vi "Sequence for 3D calibration.vi"() -> ()   [LabVIEW 2011]
doc: "The Sequence VI acquires a sequence of images and displays the images in an image control using high-level acquisition VIs. A sequence is appropriate for applications in which you want to process multiple images."
uses:
  <vilib>/userDefined/High Color/IMAQdx.ctl
  <vilib>/vision/driver/IMAQdx.llb/IMAQdx Acquisition Mode.ctl
  <vilib>/vision/driver/IMAQdx.llb/IMAQdx Buffer Number Mode.ctl
  <vilib>/vision/driver/NI_Vision_Acquisition_Software.lvlib
  Program Files/National Instruments/LabVIEW 2011/resource/objmgr/imaqdx.rc
  Program Files/Mad City Labs/NanoDrive/Madlib.dll
panel:
  out "position":dbl
  in  "Handle 2":i32
  in  "Exposure (us)":dbl(slide)=1407.017543859649 min=100.0 max=15000.0 step=100.0 scale=100.0..15000.0
  out "Acquisition  progress":i32(slide) scale=0.0..2999.0
  in  "BitsPerPixel":u32(ring) items=["Use Hardware Value"=0, "10-bit"=10, "12-bit"=12, "14-bit"=14, "16-bit"=16]
  in  "Height":u32=1080
  in  "Width":u32=1920
  in  "Number of Frames":u32=250
  in  "Frame Rate":dbl=55.0
  in  "Path":path
  in  "Camera Name":T1
  out "Image Array":T2[](array[plugin-control])
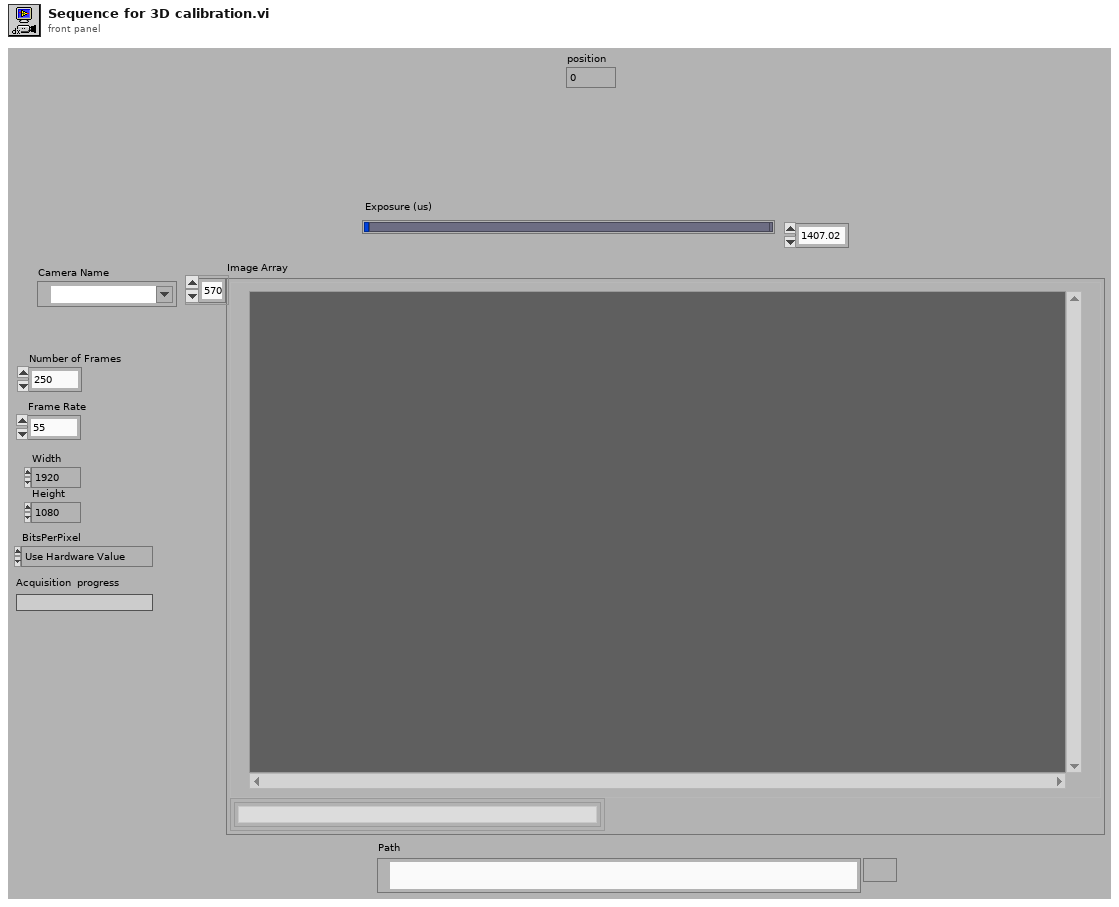
[diagram p1: front panel]
types:
  T1 = typedef "IMAQdx.ctl" = refnum<k21>
  T2 = typedef "IMAQ Image.ctl" = refnum<image>
  T3 = typedef "NI_Vision_Acquisition_Software.lvlib/IMAQdx Acquisition Mode.ctl" = enum32{"One Shot", "Continuous"}
  T4 = typedef "NI_Vision_Acquisition_Software.lvlib/IMAQdx Buffer Number Mode.ctl" = enum32{"Next", "Last", "Buffer Number"}
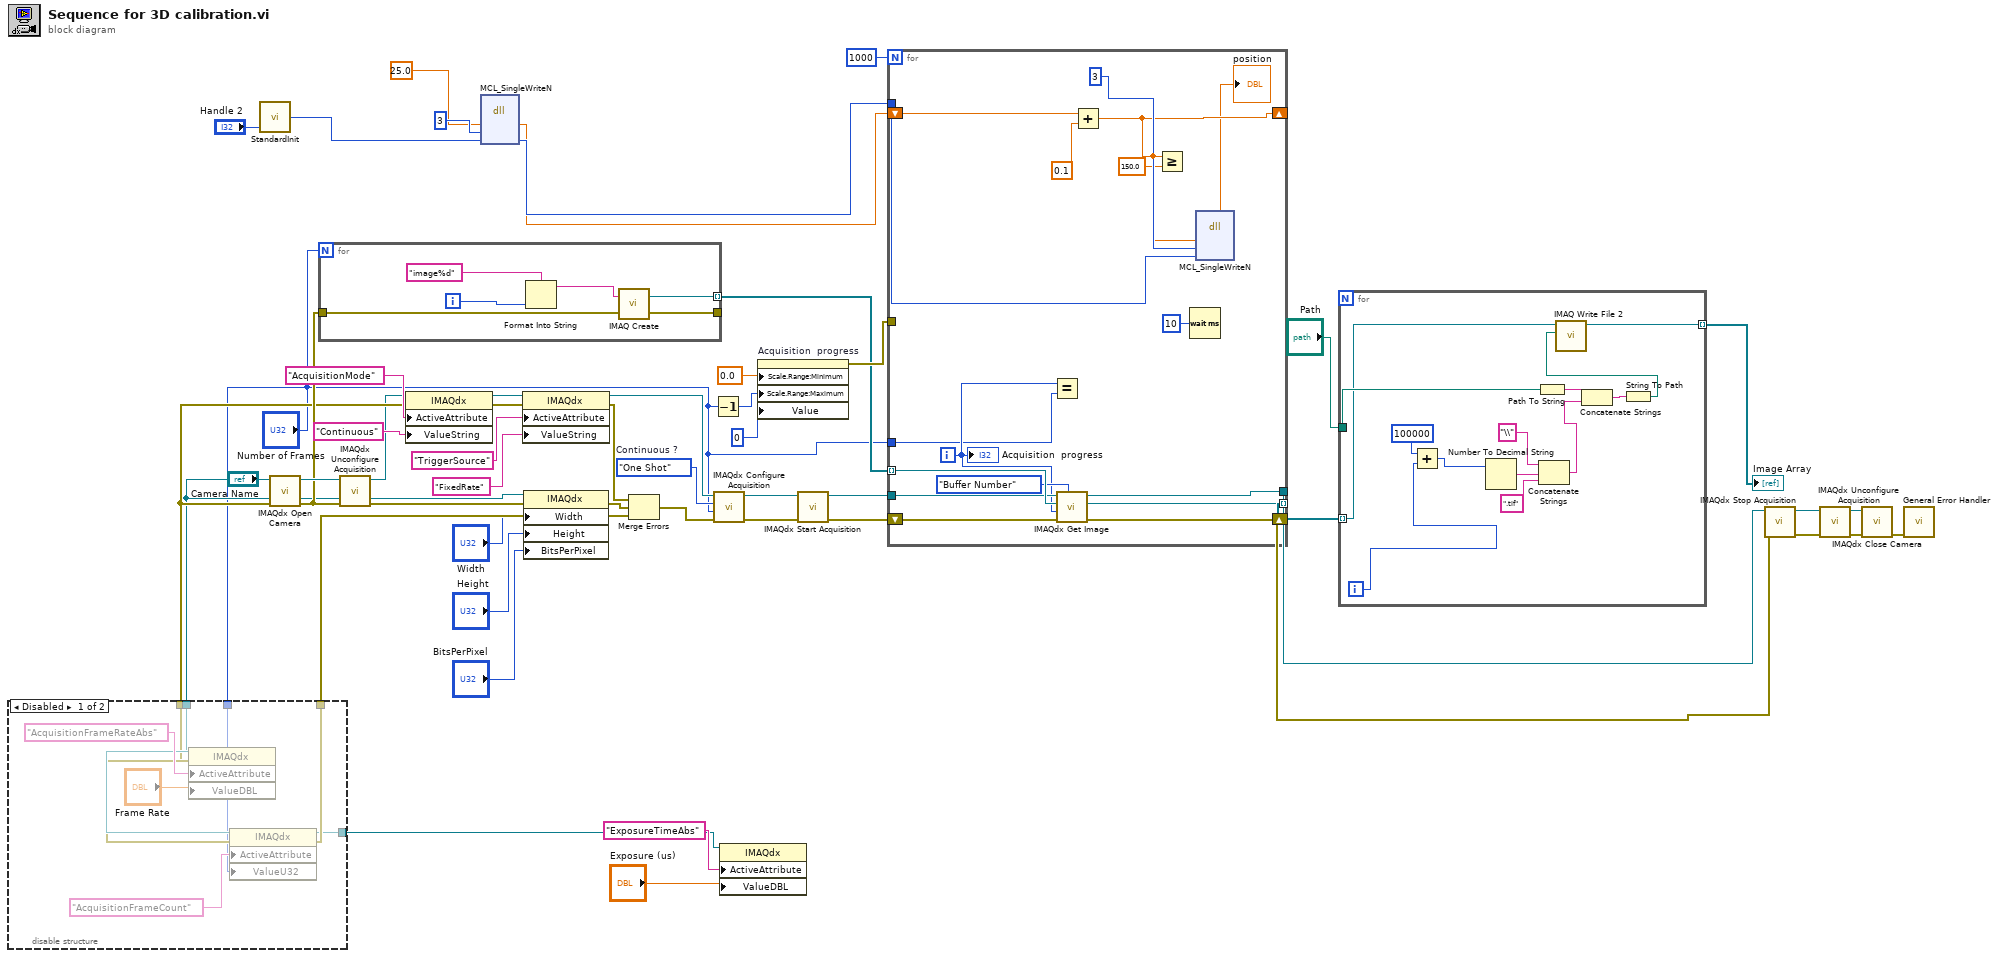
[diagram p0: block diagram]
diagram:
  w32 = IMAQdx_Acquisition_Mode."One Shot"  # Continuous ?
  n1 = call "StandardInit.vi"("Incoming Handle"="Handle 2") -> ("Outgoing Handle"=w5:i32)
  n2 = call <vilib>:"IMAQdx Open Camera.vi"("Session In"="Camera Name") -> ("error out"=w41:errorcluster, "Session Out"=w42:T1)  [unwired: 2 in, 7 out]
  n3 = for {
    N: "Number of Frames" -> [_]
    tunnel: w41 -> [w56]
    tunnel: [w55] -> w20 mode=indexing
    tunnel: [w54] -> _
    i -> [w53]
    n4 = Format Into String(format string="image%d" ("Image Name"), w53) -> (resulting string=w52:string)  [unwired: 2 in, 1 out]
    n5 = call "IMAQ Create"("Image Name"=w52, "error in (no error)"=w56) -> ("New Image"=w55:T2, "error out"=w54:errorcluster)  [unwired: 2 in, 1 out]
  }
  n6 = call <vilib>:"IMAQdx Unconfigure Acquisition.vi"("error in"=w41, "Session In"=w42) -> ("error out"=w37:errorcluster, "Session Out"=w34:T1)  [unwired: 8 out]
  n7 = disable-structure shown="Disabled" {
    disable-tunnel: [w62 _] -> w44
    disable-tunnel: w37 -> [w60 _]
    disable-tunnel: w34 -> [w59 _]
    disable-tunnel: [w58 _] -> w9
    disable-tunnel: "Number of Frames" -> [w57 _]
    frame Disabled {
      n8 = property class="IMAQdx"(reference=w59, error in=w60, "ActiveAttribute"="AcquisitionFrameRateAbs", "ValueDBL"="Frame Rate") -> (reference out=w64:T1, error out=w63:errorcluster)
      n9 = property class="IMAQdx"(reference=w64, error in=w63, "ActiveAttribute"="AcquisitionFrameCount", "ValueU32"=w57) -> (reference out=w58:T1, error out=w62:errorcluster)
    }
    frame Enabled {
    }
  }
  n10 = property class="IMAQdx"(reference=w34, error in=w37, "ActiveAttribute"="AcquisitionMode", "ValueString"="Continuous") -> (reference out=w38:T1, error out=w47:errorcluster)
  n11 = dll-call lib="C:/Program Files/Mad City Labs/NanoDrive/Madlib.dll" fn="MCL_SingleWriteN"("position"=25.0, "axis"=u32 3, "handle"=w5) -> ("position"=w2:dbl, "handle"=w3:i32)  [unwired: 4 in, 3 out]
  n12 = property class="IMAQdx"(reference=w38, error in=w47, "ActiveAttribute"="TriggerSource", "ValueString"="FixedRate") -> (reference out=w19:T1, error out=w43:errorcluster)
  n13 = property class="IMAQdx"(reference=w34, error in=w37, "Width"="Width", "Height"="Height", "BitsPerPixel"="BitsPerPixel") -> (error out=w36:errorcluster)  [unwired: 1 out]
  n14 = Merge Errors(w43, w36, w44) -> (w16:errorcluster)
  n15 = Decrement(x="Number of Frames") -> (x-1=w29:u32)
  n16 = call <vilib>:"IMAQdx Configure Acquisition.vi"("error in"=w16, "Number of Buffers"="Number of Frames", "Continuous?"=w32, "Session In"=w19) -> ("error out"=w15:errorcluster, "Session Out"=w18:T1)  [unwired: 6 out]
  n17 = property class="IMAQdx"(reference=w9, "ActiveAttribute"="ExposureTimeAbs", "ValueDBL"="Exposure (us)") -> ()  [unwired: 1 in, 2 out]
  n18 = property on="Acquisition  progress" class="Slide (strict)"("Scale.Range:Minimum"=0.0 ("Write Attribute"), "Scale.Range:Maximum"=w29, "Value"=u32 0 ("Acquisition  progress")) -> (error out=w21:errorcluster)  [unwired: 2 in, 1 out]
  n19 = call <vilib>:"IMAQdx Start Acquisition.vi"("error in"=w15, "Session In"=w18) -> ("error out"=w31:errorcluster, "Session Out"=w17:T1)  [unwired: 8 out]
  n20 = for {
    N: 1000 -> [_]
    tunnel: w20 -> [w83] mode=indexing
    shift-right: [w81] -> w28
    shift-left: w31 -> [w82]
    tunnel: [w80] -> w27
    tunnel: w17 -> [w79]
    tunnel: [w77] -> w13 mode=indexing
    tunnel: w21 -> [_]
    tunnel: "Number of Frames" -> [w75]
    tunnel: w3 -> [w71]
    shift-right: [w69] -> _
    shift-left: w2 -> [w70]
    i -> [w76]
    n21 = Equal?(x=w76, y=w75) -> ()  [unwired: 1 out]
    n22 = call <vilib>:"IMAQdx Get Image.vi"("Buffer Number Mode (Next)"=IMAQdx_Buffer_Number_Mode."Buffer Number", "error in"=w82, "Buffer Number In"=w76, "Image In"=w83, "Session In"=w79) -> ("error out"=w81:errorcluster, "Image Out"=w77:T2, "Session Out"=w80:T1)  [unwired: 4 out]
    n23 = Add(x=w70, y=0.1) -> (x+y=w69:dbl)
    n24 = Greater Or Equal?(x=w69, y=150.0) -> ()  [unwired: 1 out]
    n25 = Wait (ms)(milliseconds to wait=u32 10) -> ()  [unwired: 1 out]
    n26 = dll-call lib="C:/Program Files/Mad City Labs/NanoDrive/Madlib.dll" fn="MCL_SingleWriteN"("position"=w69, "axis"=u32 3, "handle"=w71) -> ("position"=→"position":dbl)  [unwired: 5 in, 3 out]
    "Acquisition  progress" <- w76
  }
  n27 = for {
    tunnel: "Path" -> [w86]
    tunnel: w13 -> [w85] mode=indexing
    tunnel: [w84] -> w12 mode=indexing
    i -> [w91]
    n28 = Add(x=100000, y=w91) -> (x+y=w93:i32)
    n29 = Number To Decimal String(number=w93) -> (decimal integer string=w96:string)  [unwired: 1 out]
    n30 = Path To String(path=w86) -> (string=w90:string)
    n31 = Concatenate Strings("\\" ("string"), w96, ".tif") -> (w88:string)
    n32 = Concatenate Strings(w90, w88) -> (w89:string)
    n33 = String To Path(string=w89) -> (path=w87:path)
    n34 = call-poly "IMAQ Write File 2"("File Path"=w87, "Image"=w85) -> ("Image Out (duplicate)"=w84:T2)  [unwired: 3 in, 6 out]
  }
  "Image Array" <- w12
  n35 = call <vilib>:"IMAQdx Stop Acquisition.vi"("error in"=w28, "Session In"=w27) -> ("error out"=w26:errorcluster, "Session Out"=w25:T1)  [unwired: 8 out]
  n36 = call <vilib>:"IMAQdx Unconfigure Acquisition.vi"("error in"=w26, "Session In"=w25) -> ("error out"=w24:errorcluster, "Session Out"=w23:T1)  [unwired: 8 out]
  n37 = call <vilib>:"IMAQdx Close Camera.vi"("error in"=w24, "Session In"=w23) -> ("error out"=w33:errorcluster)  [unwired: 9 out]
  n38 = call <vilib>:"General Error Handler.vi"("error in (no error)"=w33) -> ()  [unwired: 1 in, 14 out]
